vi "2. Class and Interface Coercion Rules.vi"   [LabVIEW 2023]
doc: "This VI demonstrates the type coercion rules for LabVIEW classes and interfaces."
uses:
  Lever/Lever.lvclass
  Nailer/Nailer.lvclass
  c:/dev/_r/4/eng/lv-core/lvpostprocessingd/lv_mc_x86_64/dist_i386/examples/Object-Oriented Programming/Basic Interfaces/Lever/Lever.lvclass
  Flathead/Flathead.lvclass
  Box/Box.lvclass
  House Key/House Key.lvclass
  c:/dev/_r/4/eng/lv-core/lvpostprocessingd/lv_mc_x86_64/dist_i386/examples/Object-Oriented Programming/Basic Interfaces/Tool/Tool.lvclass
  Tool/Tool.lvclass
panel:
  # "Overview: Demonstrates the type coercion rules for LabVIEW classes and interfaces.\nInstructions:\nOpen the block diagram and refer to the comments there."
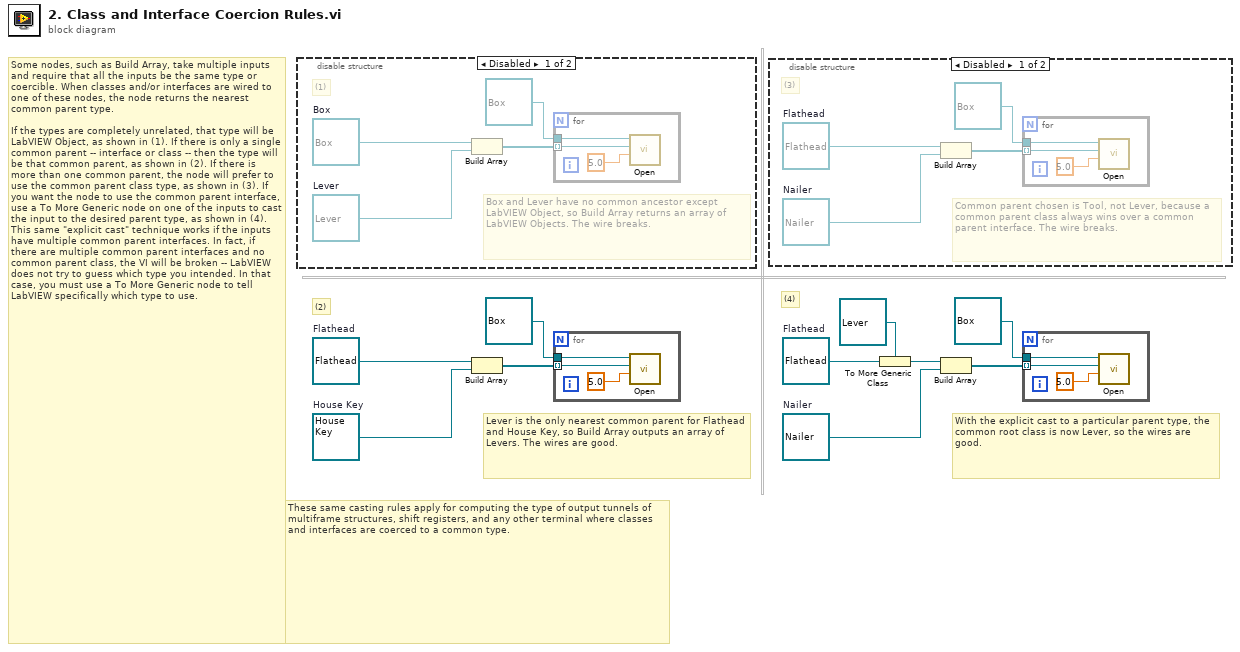
[diagram p0: block diagram]
diagram:
  w1 = refnum<class "House Key.lvclass"> refnum  # House Key
  w2 = refnum<class "Flathead.lvclass"> refnum  # Flathead
  w8 = refnum<class "Nailer.lvclass"> refnum  # Nailer
  w7 = refnum<class "Flathead.lvclass"> refnum  # Flathead
  # "These same casting rules apply for computing the type of output tunnels of multiframe structures, shift registers, and any other terminal where classes and interfaces are coerced to a common type."
  # "(4)"
  # "(2)"
  # "Lever is the only nearest common parent for Flathead and House Key, so Build Array outputs an array of Levers. The wires are good."
  # "Some nodes, such as Build Array, take multiple inputs and require that all the inputs be the same type or coercible. When classes and/or interfaces are wired to one of these nodes, the node returns the nearest common parent type. \n\nIf the types are completely unrelated, that type will be LabVIEW Object, as shown in (1). If there is only a single common parent -- interface or class -- then the type will be that common parent, as shown in (2). If there is more than one common parent, the node will prefer to use the common parent class type, as shown in (3). If you want the node to use the common parent interface, use a To More Generic node on one of the inputs to cast the input to the desired parent type, as shown in (4). This same \"explicit cast\" technique works if the inputs have multiple common parent interfaces. In fact, if there are multiple common parent interfaces and no common parent class, the VI will be broken -- LabVIEW does not try to guess which type you intended. In that case, you must use a To More Generic node to tell LabVIEW specifically which type to use."
  # "With the explicit cast to a particular parent type, the common root class is now Lever, so the wires are good."
  n1 = disable-structure shown="Disabled" {
    frame Disabled {
      w11 = refnum<class "Lever.lvclass"> refnum  # Lever
      w12 = refnum<class "Box.lvclass"> refnum  # Box
      # "(1)"
      # "Box and Lever have no common ancestor except LabVIEW Object, so Build Array returns an array of LabVIEW Objects. The wire breaks."
      n2 = Build Array(w12, w11) -> (w13:refnum<class>[])
      n3 = for {
        tunnel: refnum<class "Box.lvclass"> refnum ("Box.lvclass") -> [w17]
        tunnel: w13 -> [w16] mode=indexing
        n4 = call "Open.vi"("force"=5.0, "Lever"=w16, "Box in"=w17) -> ()  [unwired: 8 in, 1 out]
      }
    }
    frame Enabled {
    }
  }
  n5 = Build Array(w2, w1) -> (w4:refnum<class "Lever.lvclass">[])
  n6 = for {
    tunnel: refnum<class "Box.lvclass"> refnum ("Box.lvclass") -> [w20]
    tunnel: w4 -> [w19] mode=indexing
    n7 = call "Open.vi"("force"=5.0, "Lever"=w19, "Box in"=w20) -> ()  [unwired: 8 in, 1 out]
  }
  n8 = disable-structure shown="Disabled" {
    frame Disabled {
      w23 = refnum<class "Nailer.lvclass"> refnum  # Nailer
      w24 = refnum<class "Flathead.lvclass"> refnum  # Flathead
      # "(3)"
      # "Common parent chosen is Tool, not Lever, because a common parent class always wins over a common parent interface. The wire breaks."
      n9 = Build Array(w24, w23) -> (w22:refnum<class "Tool.lvclass">[])
      n10 = for {
        tunnel: refnum<class "Box.lvclass"> refnum ("Box.lvclass") -> [w27]
        tunnel: w22 -> [w26] mode=indexing
        n11 = call "Open.vi"("force"=5.0, "Lever"=w26, "Box in"=w27) -> ()  [unwired: 8 in, 1 out]
      }
    }
    frame Enabled {
    }
  }
  n12 = To More Generic Class(target class=refnum<class "Lever.lvclass"> refnum ("Lever.lvclass"), reference=w7) -> (generic class reference=w6:refnum<class "Lever.lvclass">)
  n13 = Build Array(w6, w8) -> (w9:refnum<class "Lever.lvclass">[])
  n14 = for {
    tunnel: refnum<class "Box.lvclass"> refnum ("Box.lvclass") -> [w30]
    tunnel: w9 -> [w29] mode=indexing
    n15 = call "Open.vi"("force"=5.0, "Lever"=w29, "Box in"=w30) -> ()  [unwired: 8 in, 1 out]
  }
